vi "CollectDataQueue.vi"(1 "ChannelArryRead":bool[](array[boolean])) -> (15 "CollectDataQueue":refnum<queue>)   [LabVIEW 2020, in "NI_DAQ.lvclass"]
uses:
  NI_DAQ.lvclass
  E:/01_Project/CXXXX/GKN/C18726_27program_191115004/software/DAQ/DAQ_operation_type.ctl
panel:
  out "波形图":dbl[][](graph)
  # "0手动\n1自动1阶段\n2自动2阶段"
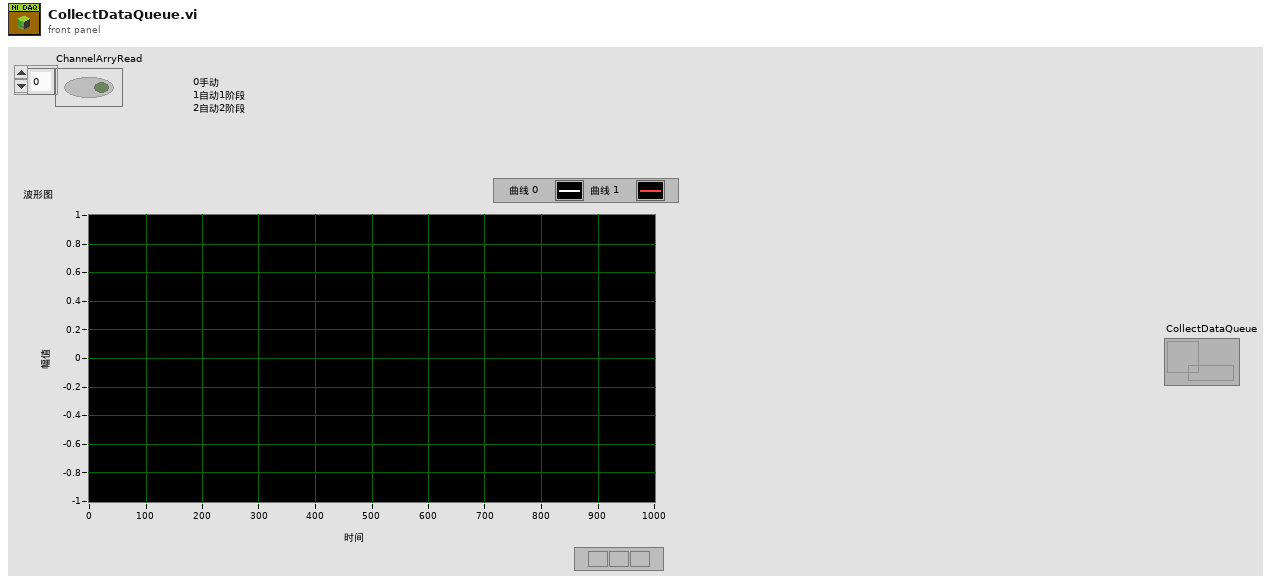
[diagram p1: front panel]
types:
  T1 = typedef "DAQ_operation_type.ctl" = enum16{"idle", "read", "write", "clear", "init", "destroy"}
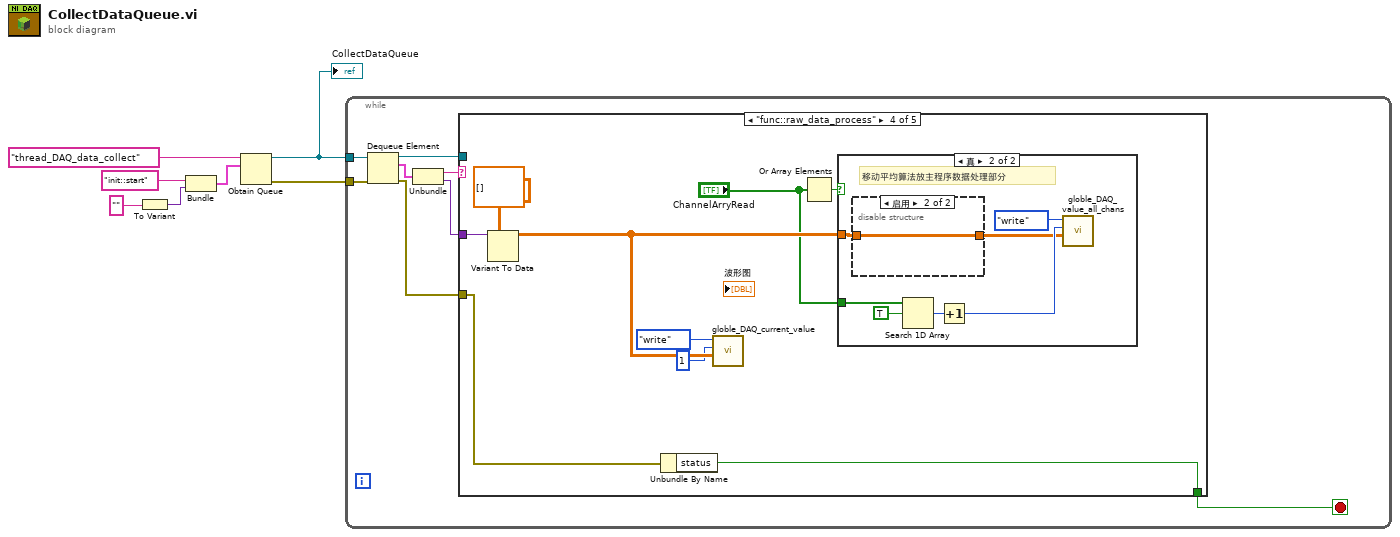
[diagram p0: block diagram]
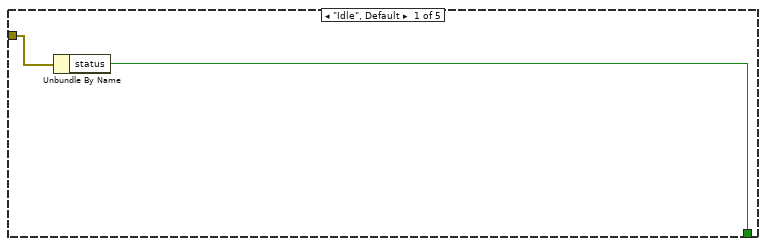
[diagram p2: hidden frame]
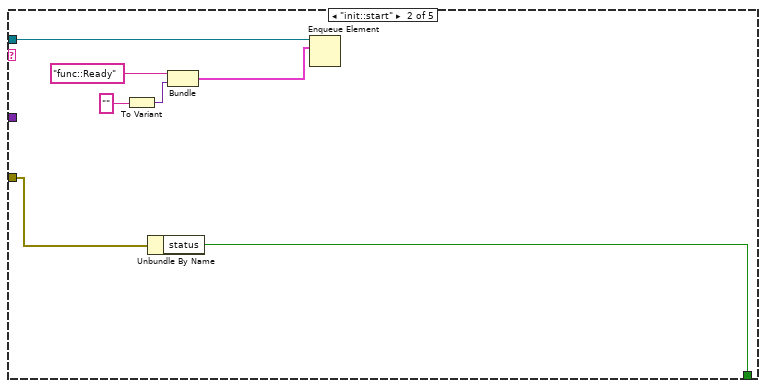
[diagram p3: hidden frame]
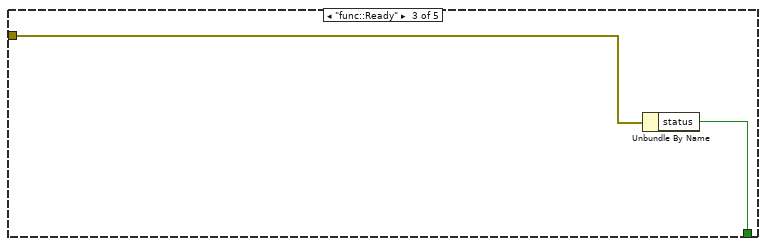
[diagram p4: hidden frame]
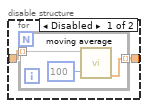
[diagram p6: hidden frame]
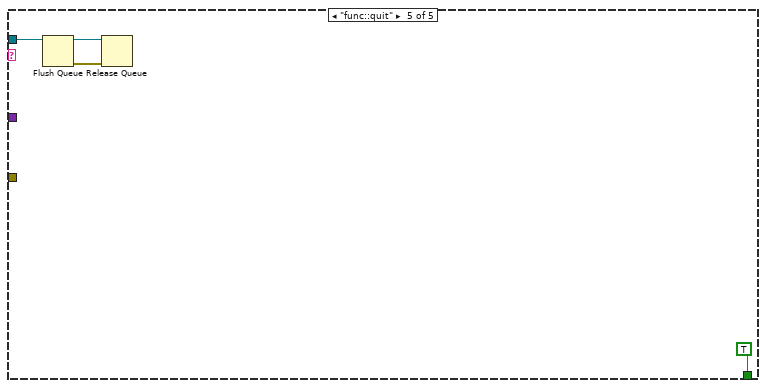
[diagram p7: hidden frame]
diagram:
  n1 = To Variant(anything="") -> (Variant=w6:variant)
  n2 = Bundle("init::start", "Variant"=w6) -> (w4:cluster{string, "Variant":variant})  [unwired: 1 in]
  n3 = Obtain Queue(name (unnamed)="thread_DAQ_data_collect" ("名称（未命名）"), element data type=w4) -> (queue out=w3:refnum<queue>, error out=w2:errorcluster)  [unwired: 3 in, 1 out]
  "CollectDataQueue" <- w3
  n4 = while {
    tunnel: w3 -> [w14]
    tunnel: w2 -> [w13]
    stop <- w9 stop-if-true
    n5 = Dequeue Element(queue=w14, error in (no error)=w13) -> (queue out=w10:refnum<queue>, element=w15:cluster{string, "Variant":variant}, error out=w8:errorcluster)  [unwired: 1 in, 1 out]
    n6 = Unbundle(w15) -> (w12:string, "Variant"=w11:variant)
    n7 = case shown="\"func::raw_data_process\"" w12 {
      tunnel: w11 -> [_ _ _ w35 _]
      tunnel: w10 -> [_ w24 _ _ w50]
      tunnel: [w16 w18 w25 w33 TRUE] -> w9
      tunnel: w8 -> [w17 w19 w26 w34 _]
      frame "Idle", Default {
        n8 = Unbundle By Name(w17) -> ("status"=w16:bool)
      }
      frame "init::start" {
        n9 = To Variant(anything="") -> (Variant=w21:variant)
        n10 = Unbundle By Name(w19) -> ("status"=w18:bool)
        n11 = Bundle("func::Ready", "Variant"=w21) -> (w20:cluster{string, "Variant":variant})  [unwired: 1 in]
        n12 = Enqueue Element(queue=w24, element=w20) -> ()  [unwired: 2 in, 3 out]
      }
      frame "func::Ready" {
        n13 = Unbundle By Name(w26) -> ("status"=w25:bool)
      }
      frame "func::raw_data_process" {
        n14 = Variant To Data(type=dbl[][] [] ("波形图"), Variant=w35) -> (data=w31:dbl[][])  [unwired: 1 in, 1 out]
        n15 = Unbundle By Name(w34) -> ("status"=w33:bool)
        n16 = call "globle_DAQ_current_value.vi"("data in"=w31, "chanel_nbr"=1, "opearte"=DAQ_operation_type."write") -> ()  [unwired: 7 in, 2 out]
        n17 = Or Array Elements(Boolean array="ChannelArryRead") -> (logical OR=w28:bool)
        n18 = case shown="真" w28 {
          tunnel: w31 -> [_ w41]
          tunnel: "ChannelArryRead" -> [_ w38]
          frame False {
          }
          frame True {
            # "移动平均算法放主程序数据处理部分"
            n19 = disable-structure shown="启用" {
              disable-tunnel: w41 -> [w44 w48]
              disable-tunnel: [w43 w48] -> w36
              frame Disabled {
                n20 = for {
                  tunnel: w44 -> [w47] mode=indexing
                  tunnel: [w45] -> w43 mode=indexing
                  n21 = call "moving average.vi"("Num"=100, "Filtered X"=w47) -> ("数组 2"=w45:dbl[])  [unwired: 9 in]
                }
              }
              frame Enabled {
              }
            }
            n22 = Search 1D Array(1D array=w38, element=TRUE) -> (index of element=w39:i32)  [unwired: 1 in]
            n23 = Increment(x=w39) -> (x+1=w37:i32)
            n24 = call "globle_DAQ_value_all_chans.vi"("data_in"=w36, "chanel_nbr"=w37, "opearte"=DAQ_operation_type."write") -> ()  [unwired: 6 in, 3 out]
          }
        }
      }
      frame "func::quit" {
        n25 = Flush Queue(queue=w50) -> (queue out=w51:refnum<queue>, error out=w52:errorcluster)  [unwired: 1 in, 1 out]
        n26 = Release Queue(queue=w51, error in (no error)=w52) -> ()  [unwired: 1 in, 3 out]
      }
    }
  }
